vi "Set Gain.vi"(8 "error in (no error)":errorcluster, 10 "Gain":u8 step=1, 11 "Inovance_Camera in":refnum<class "Inovance_Camera.lvclass">) -> (0 "error out":errorcluster, 3 "Inovance_Camera out":refnum<class "Inovance_Camera.lvclass">)   [LabVIEW 2023, in "Inovance_Camera.lvlib" / "Inovance_Camera.lvclass"]
uses:
  Inovance_Camera.lvclass
  C:/Program Files/National Instruments/LabVIEW 2023/vi.lib/ActorFramework/Actor/Actor.lvclass
  <vilib>/userDefined/High Color/IMAQdx.ctl
  Inovance_Camera.lvclass/Inovance_Camera.ctl
  <vilib>/ActorFramework/Actor/Actor.lvclass/Actor.ctl
  Interfaces/AbstractInstrumentClasses/Cameras_LV/CameraComm Messages/Gain Set Msg/Gain Set Msg.lvclass/Gain Set Msg.ctl
  <vilib>/ActorFramework/Message Enqueuer/Message Enqueuer.lvclass/Message Enqueuer.ctl
  <vilib>/ActorFramework/Message Enqueuer/Enqueue.vi
  Interfaces/AbstractInstrumentClasses/Cameras_LV/CameraComm Messages/Gain Set Msg/Gain Set Msg.lvclass
  C:/Program Files/National Instruments/LabVIEW 2023/vi.lib/ActorFramework/Message/Message.lvclass
  <vilib>/ActorFramework/Message Priority Queue/Priority Enqueue.vi
  Inovance_Camera.lvlib
  <vilib>/ActorFramework/Actor/Actor.lvclass
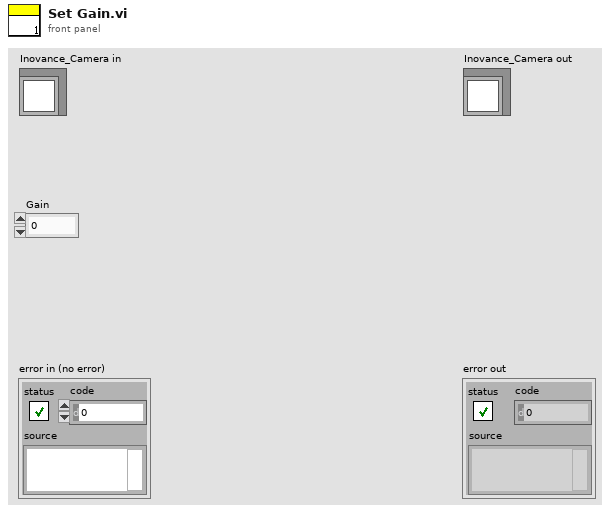
[diagram p1: front panel]
types:
  T1 = typedef "IMAQdx.ctl" = refnum<k21>
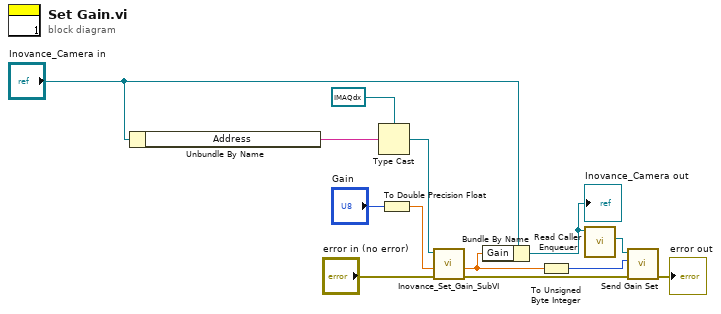
[diagram p0: block diagram]
diagram:
  n1 = Unbundle By Name("Inovance_Camera in") -> ("Address"=w4:string)
  n2 = Type Cast(type=T1 refnum ("Refnum out"), x=w4) -> (*(type *) &x=w2:T1)
  n3 = To Double Precision Float(number="Gain") -> (double precision float=w13:dbl)
  n4 = call "Inovance_Set_Gain_SubVI.vi"("error in (no error)"="error in (no error)", "Gain"=w13, "Refnum in"=w2) -> ("error out"=w9:errorcluster, "Gain Out"=w7:dbl)  [unwired: 6 in, 1 out]
  n5 = Bundle By Name(cluster="Inovance_Camera in", "Gain"=w7) -> (w1:refnum<class "Inovance_Camera.lvclass">)
  "Inovance_Camera out" <- w1
  n6 = To Unsigned Byte Integer(number=w7) -> (unsigned 8bit integer=w6:u8)
  n7 = call <vilib>:"Read Caller Enqueuer.vi"("Actor"=w1) -> ("Caller Enqueuer"=w10:refnum<class "Message Enqueuer.lvclass">)  [unwired: 10 in]
  n8 = call "Send Gain Set.vi"("error in (no error)"=w9, "Gain"=w6, "Message Enqueuer"=w10) -> ("error out"=→"error out":errorcluster)  [unwired: 7 in, 1 out]
